vi "Test Test Unit API.vi"() -> ()   [LabVIEW 2025]
doc: "Test Unit API Tester."
uses:
  Test Unit.lvlib
  <vilib>/Utility/error.llb/DialogType.ctl
  <vilib>/Test Bench Framework/Test Executive.lvlibp/TestEngine/TestEngine/TestEngine/Report Format.ctl
  <vilib>/Test Bench Framework/Test Executive.lvlibp/TestEngine/TestEngine/TestEngine/Test Engine.lvclass
  <vilib>/Test Bench Framework/Test Executive.lvlibp/TestEngine/TestEngine/TestEngine/Typedefs/Local Report Configuration.ctl
  <vilib>/Test Bench Framework/Test Executive.lvlibp/TestEngine/TestEngine/TestEngine/Typedefs/Database Configuration.ctl
  <vilib>/Test Bench Framework/Test Executive.lvlibp/TestEngine/TestEngine/TestEngine/Typedefs/TestEngine Cofiguration.ctl
panel:
  in  "LanguageChanged":bool
  in  "Tab Control":T1(tab)
  in  "Number of socket":i32=1 min=1 max=255 step=1
  in  "TitleWindows":bool
  in  "Run New Module":bool
  in  "Select Module":i32(ring)=-1 caption="Select Module\nTo send Request to" items=["All"=-1]
  in  "Refresh Modules":bool
  in  "TestEngine Cofiguration":T2={"Break on Failure"=FALSE, "Automatically handle TestVI error"={"Enable"=FALSE, "Handle"=enum."Termination test"}, "Local Report Configuration"={"Report Folder Path"=path "D:/", "Format"=enum."CSV(,)", "Disable"=FALSE, "Build Date Folder?"=TRUE, "Execl Template Path"=path ""}, "Database Configuration"={"Connection String Expression"="", "Microsoft Data Link File"=path "", "Connection Type"=enum."Use Connection String Expression", "Enable"=FALSE}, "Ignore breakpoint"=FALSE, "Filter Result"=FALSE}
  in  "Cofiguration":bool
  in  "Load Sequence":bool
  in  "File Path Control":path
  in  "Set SN":bool
  in  "Socket":i32
  in  "Serial Number":string
  in  "Abort VI":bool=TRUE
  in  "Terminate Test":bool
  in  "Start UUTsTest":bool
  in  "Start Test":bool
  in  "Test Socket":i32
  in  "Enable Socket":bool[](array[boolean])
  in  "Set Variable":bool
  in  "Get Variable":bool
  in  "Socket(Variable)":i32
  in  "Variable Name":string
  out "Value":variant
  out "last error":errorcluster
  out "Active Modules":string[](array[string])
  in  "Stop Module":bool
  out "Status":string
  # "启动单槽位测试"
  # "启动多槽位测试"
  # "只有这个模式可以使用同步属性"
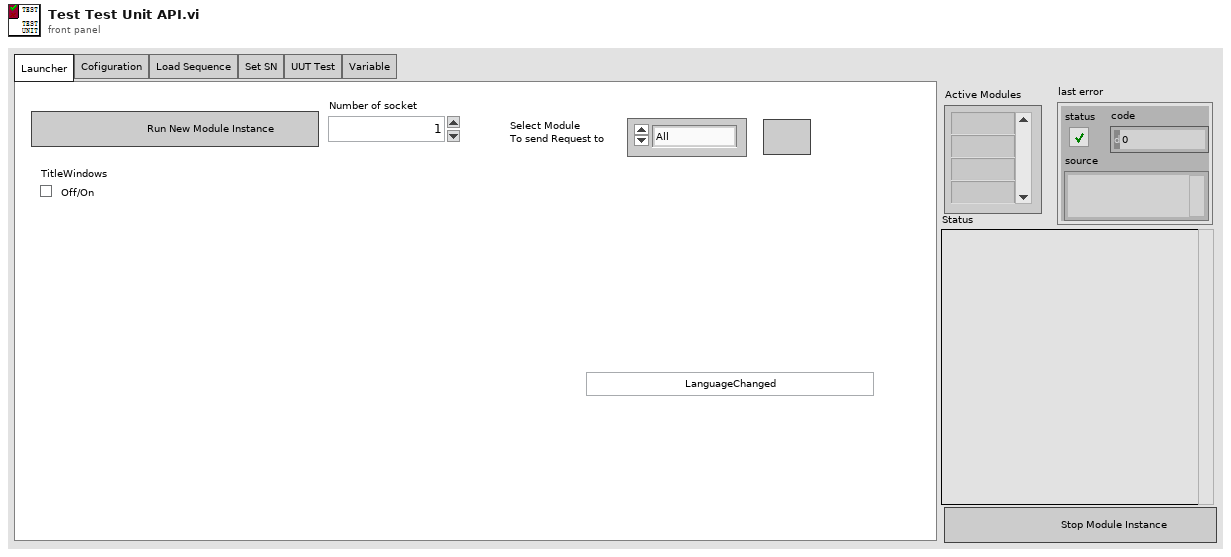
[diagram p1: front panel]
types:
  T1 = enum32{"Launcher", "Cofiguration", "Load Sequence", "Set SN", "UUT Test", "Variable"}
  T2 = typedef "Test Executive.lvlibp/Test Engine.lvlib/Test Engine.lvclass/TestEngine Cofiguration.ctl" = cluster{"Break on Failure":bool, "Automatically handle TestVI error":cluster{"Enable":bool, "Handle":enum16{"Termination test", "Ignore error"}}, "Local Report Configuration":T3, "Database Configuration":T5, "Ignore breakpoint":bool, "Filter Result":bool}
  T3 = typedef "Test Executive.lvlibp/Test Engine.lvlib/Test Engine.lvclass/Local Report Configuration.ctl" = cluster{"Report Folder Path":path, "Format":T4, "Disable":bool, "Build Date Folder?":bool, "Execl Template Path":path}
  T4 = typedef "Test Executive.lvlibp/Test Engine.lvlib/Test Engine.lvclass/Report Format.ctl" = enum16{"Excel", "CSV(Tab)", "CSV(,)", "CSV(;)", "TEXT", "HTML"}
  T5 = typedef "Test Executive.lvlibp/Test Engine.lvlib/Test Engine.lvclass/Database Configuration.ctl" = cluster{"Connection String Expression":string, "Microsoft Data Link File":path, "Connection Type":enum16{"Use Connection String Expression", "Use Microsoft Data Link File"}, "Enable":bool}
  T6 = typedef "Test Unit.lvlib/Broadcast Events--cluster.ctl" = cluster{"Module Did Init":refnum<user-event>, "Status Updated":refnum<user-event>, "Error Reported":refnum<user-event>, "Module Did Stop":refnum<user-event>, "Update Module Execution Status":refnum<user-event>}
  T7 = typedef "DialogType.ctl" = u16
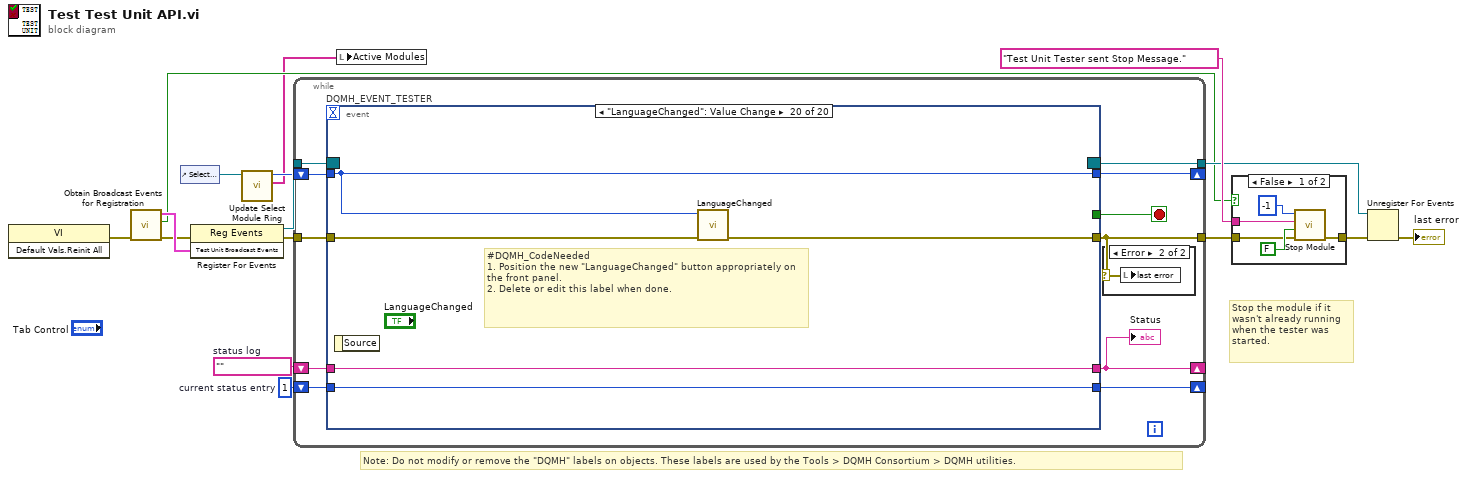
[diagram p0: block diagram]
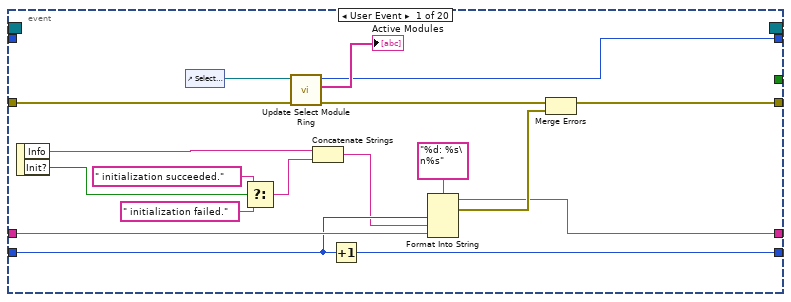
[diagram p4: hidden frame]
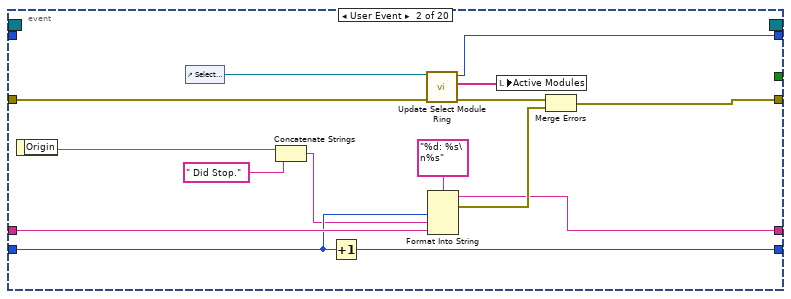
[diagram p5: hidden frame]
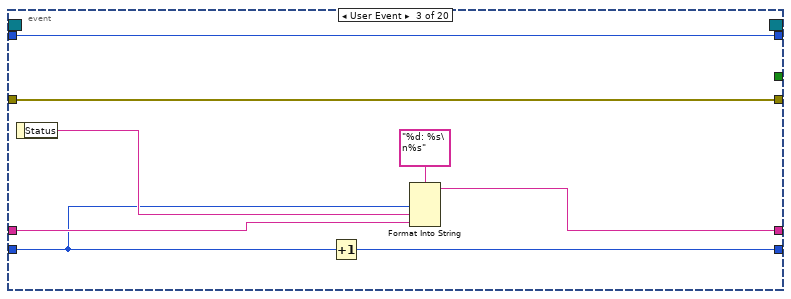
[diagram p6: hidden frame]
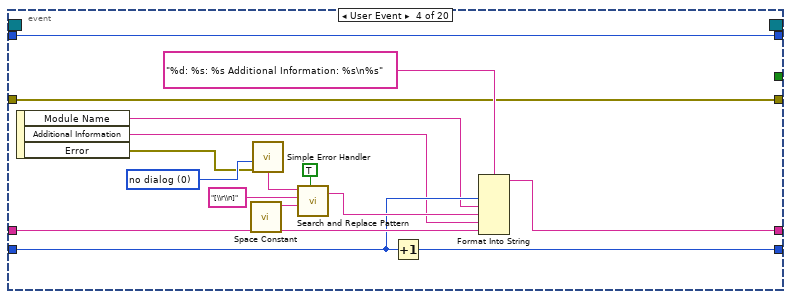
[diagram p7: hidden frame]
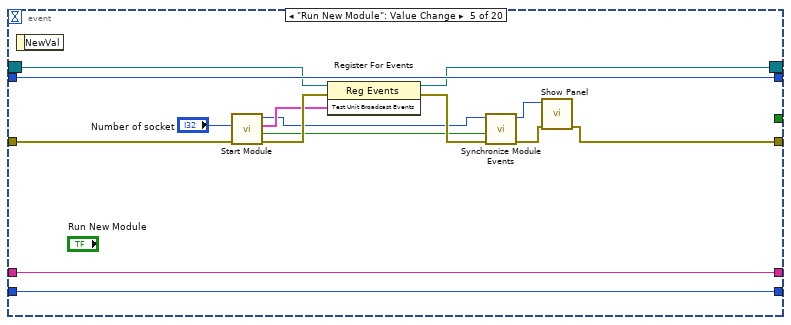
[diagram p8: hidden frame]
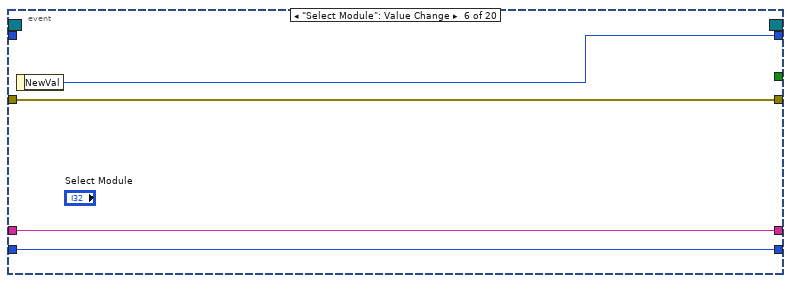
[diagram p9: hidden frame]
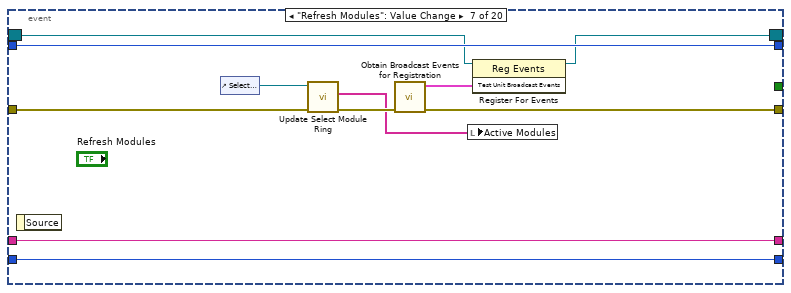
[diagram p10: hidden frame]
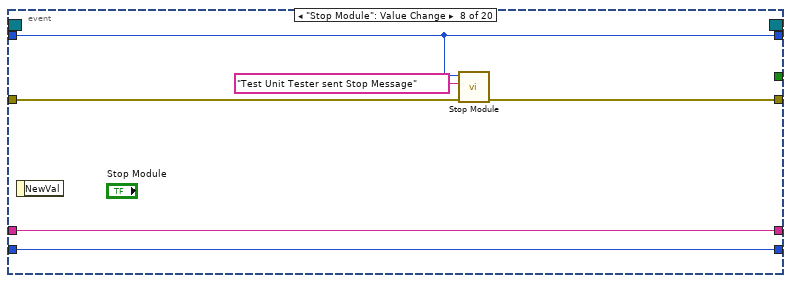
[diagram p11: hidden frame]
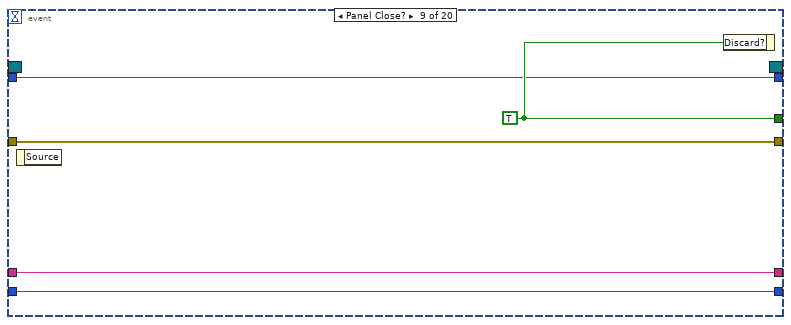
[diagram p12: hidden frame]
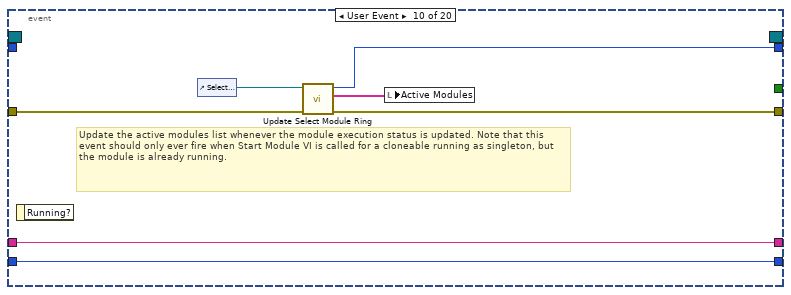
[diagram p13: hidden frame]
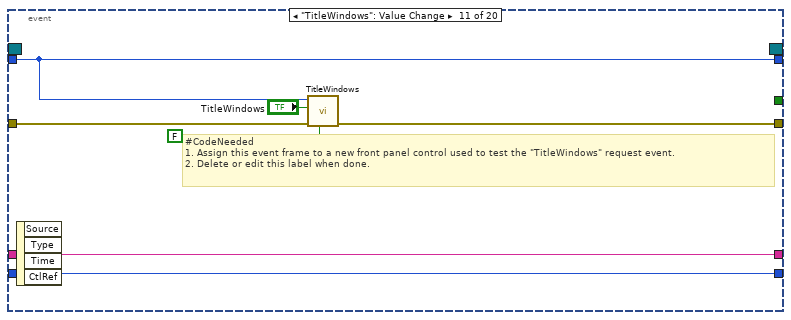
[diagram p14: hidden frame]
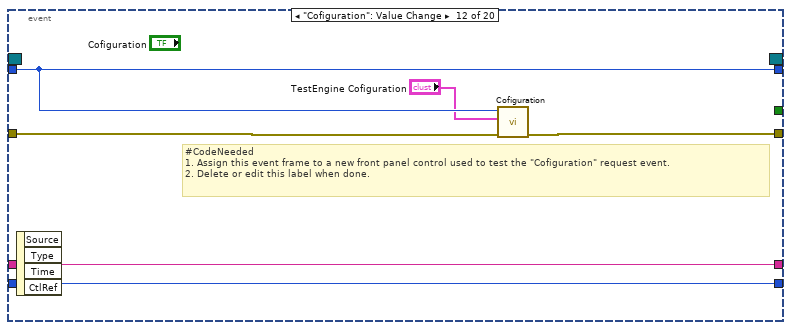
[diagram p15: hidden frame]
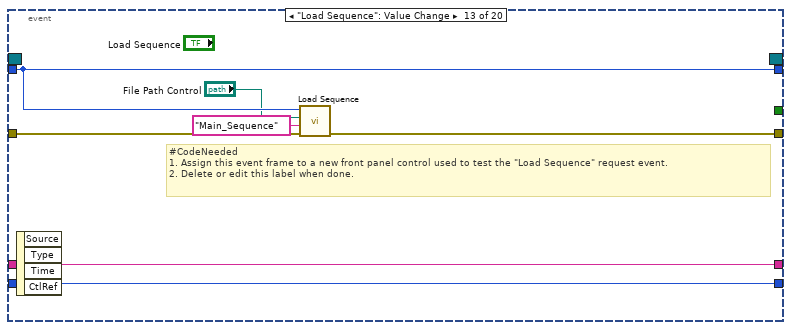
[diagram p16: hidden frame]
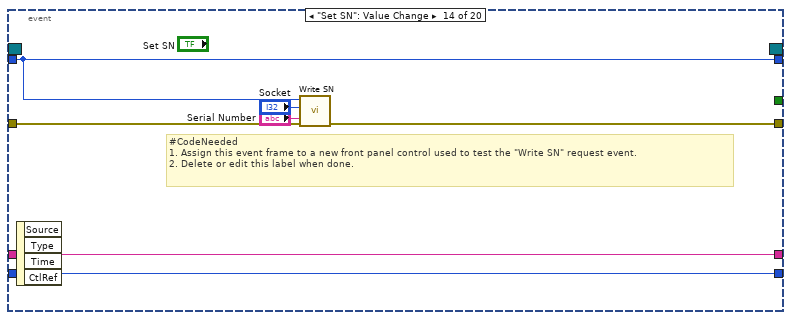
[diagram p17: hidden frame]
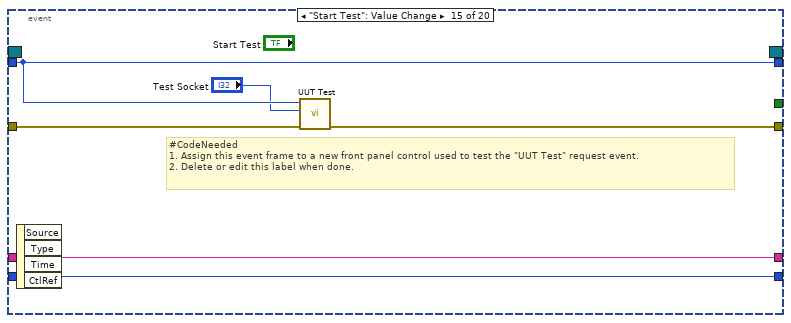
[diagram p18: hidden frame]
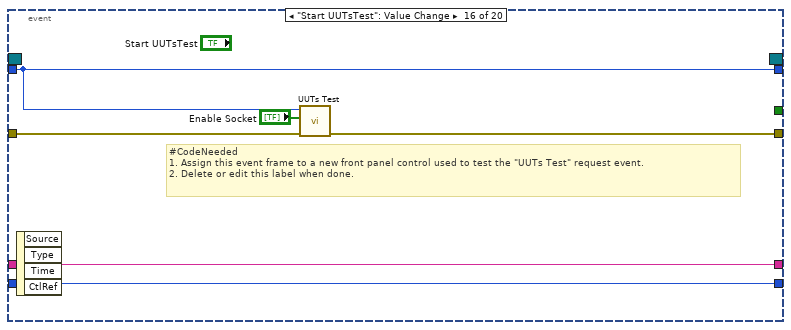
[diagram p19: hidden frame]
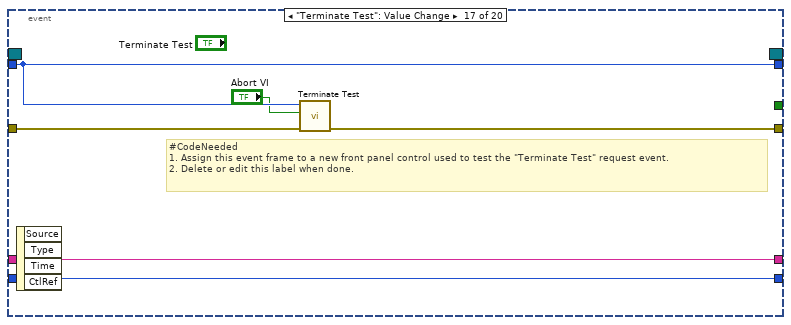
[diagram p20: hidden frame]
diagram:
  w13 = 1  # current status entry
  w14 = ""  # status log
  # "Stop the module if it wasn't already running when the tester was started."
  # "Note: Do not modify or remove the \"DQMH\" labels on objects. These labels are used by the Tools > DQMH Consortium > DQMH utilities."
  n1 = invoke class="VI" method="Default Vals.Reinit All"() -> (error out=w8:errorcluster)  [unwired: 3 in, 2 out]
  n2 = call "Obtain Broadcast Events for Registration.vi"("error in"=w8) -> ("error out"=w7:errorcluster, "Already running?"=w6:bool, "Test Unit Broadcast Events"=w12:T6)  [unwired: 8 in]
  n3 = control-ref of="Select Module"() -> (w3:refnum<vi>)
  n4 = register-events(error in=w7, w12) -> (reference out=w16:refnum<event-registration>, error out=w11:errorcluster)  [unwired: 1 in]
  n5 = call "Update Select Module Ring.vi"("Select Module Ring Ref"=w3) -> ("Active Modules (Array)"=w1:string[], "New Module Ring Value"=w2:i32)  [unwired: 8 in, 1 out]
  n6 = while {
    tunnel: w16 -> [w27]
    tunnel: [w18] -> w5
    tunnel: w11 -> [w26]
    shift-right: [w22] -> _
    shift-left: w14 -> [w24]
    shift-right: [w23] -> _
    shift-left: w13 -> [w25]
    shift-right: [w20] -> _
    shift-left: w2 -> [w21]
    tunnel: [w19] -> w9
    stop <- w17 stop-if-true
    n7 = event "DQMH_EVENT_TESTER" shown="[19] \"LanguageChanged\": Value Change" {
      selector: w27 -> [_ _ _ _ w94 _ w110 _ _ _ _ _ _ _ _ _ _ _ _ _]
      dyn-events: [_ _ _ _ w93 _ w109 _ _ _ _ _ _ _ _ _ _ _ _ _] -> w19
      timeout: _ -> [_ _ _ _ _ _ _ _ _ _ _ _ _ _ _ _ _ _ _ _]
      tunnel: [_ _ _ _ _ _ _ _ w126 _ _ _ _ _ _ _ _ _ _ _] -> w17
      tunnel: [w36 w53 w69 w73 w86 w104 w106 w117 w125 w129 w136 w142 w149 w156 w162 w168 w174 w179 w191 w196] -> w18
      tunnel: w26 -> [w38 w55 w69 w73 w95 w104 w111 w118 w125 w130 w140 w146 w153 w160 w166 w172 w178 w183 w195 w200]
      tunnel: w25 -> [w43 w58 w62 w76 w97 w102 w114 w120 w123 w132 w138 w144 w151 w158 w164 w170 w176 w181 w193 w198]
      tunnel: w24 -> [w44 w59 w65 w77 w98 w103 w115 w121 w124 w133 w139 w145 w152 w159 w165 w171 w177 w182 w194 w199]
      tunnel: [w41 w56 w66 w75 w98 w103 w115 w121 w124 w133 w139 w145 w152 w159 w165 w171 w177 w182 w194 w199] -> w22
      tunnel: [w42 w57 w68 w74 w97 w102 w114 w120 w123 w132 w138 w144 w151 w158 w164 w170 w176 w181 w193 w198] -> w23
      tunnel: w21 -> [_ _ w63 w85 w96 _ w113 w119 w122 _ w137 w143 w150 w157 w163 w169 w175 w180 w192 w197]
      tunnel: [w33 w50 w63 w85 w96 w101 w113 w119 w122 w128 w137 w143 w150 w157 w163 w169 w175 w180 w192 w197] -> w20
      event User Event {
        n8 = event-data() -> ("Info"=w40:string, "Init?"=w30:bool)  [unwired: 1 in]
        n9 = control-ref of="Select Module"() -> (w35:refnum<vi>)
        n10 = Select(t=" initialization succeeded.", s=w30, f=" initialization failed.") -> (s? t:f=w29:string)
        n11 = call "Update Select Module Ring.vi"("error in"=w38, "Select Module Ring Ref"=w35) -> ("error out"=w37:errorcluster, "Active Modules (Array)"=→"Active Modules":string[], "New Module Ring Value"=w33:i32)  [unwired: 7 in]
        n12 = Concatenate Strings(w40, w29) -> (w39:string)
        n13 = Increment(x=w43) -> (x+1=w42:i32)
        n14 = Format Into String(format string="%d: %s\n%s", w43, w39, w44) -> (resulting string=w41:string, error out=w46:errorcluster)  [unwired: 2 in]
        n15 = Merge Errors(w37, w46) -> (w36:errorcluster)
      }
      event User Event {
        n16 = event-data() -> ("Origin"=w48:string)  [unwired: 1 in]
        n17 = control-ref of="Select Module"() -> (w52:refnum<vi>)
        n18 = Concatenate Strings(w48, " Did Stop.") -> (w47:string)
        n19 = Increment(x=w58) -> (x+1=w57:i32)
        n20 = call "Update Select Module Ring.vi"("error in"=w55, "Select Module Ring Ref"=w52) -> ("error out"=w54:errorcluster, "Active Modules (Array)"=w51:string[], "New Module Ring Value"=w50:i32)  [unwired: 7 in]
        n21 = Format Into String(format string="%d: %s\n%s", w58, w47, w59) -> (resulting string=w56:string, error out=w61:errorcluster)  [unwired: 2 in]
        n22 = local write "Active Modules"(w51) -> ()
        n23 = Merge Errors(w54, w61) -> (w53:errorcluster)
      }
      event User Event {
        n24 = event-data() -> ("Status"=w64:string)  [unwired: 1 in]
        n25 = Increment(x=w62) -> (x+1=w68:i32)
        n26 = Format Into String(format string="%d: %s\n%s", w62, w64, w65) -> (resulting string=w66:string)  [unwired: 2 in, 1 out]
      }
      event User Event {
        w78 = T7 0 items=["no dialog", "OK message", "continue or stop message", "OK message + warnings", "continue/stop + warnings"] ("type of dialog (OK msg:1)")
        n27 = event-data() -> ("Module Name"=w72:string, "Additional Information"=w71:string, "Error"=w70:errorcluster)  [unwired: 1 in]
        n28 = call <vilib>:"Space Constant.vi"() -> ("String"=w82:string)
        n29 = call <vilib>:"Simple Error Handler.vi"("type of dialog (OK msg:1)"=w78, "error in (no error)"=w70) -> ("message"=w79:string)  [unwired: 3 in, 4 out]
        n30 = call <vilib>:"Search and Replace Pattern.vi"("string"=w79, "regular expression (\"\")"="[\\r\\n]" ("regular expression (\"\")"), "replace string (\"\")"=w82, "replace all? (F)"=TRUE ("replace all CR/LF with spaces")) -> ("result string"=w80:string)  [unwired: 1 in, 1 out]
        n31 = Increment(x=w76) -> (x+1=w74:i32)
        n32 = Format Into String(format string="%d: %s: %s Additional Information: %s\n%s", w76, w72, w80, w71, w77) -> (resulting string=w75:string)  [unwired: 2 in, 1 out]
      }
      event "Run New Module": Value Change {
        n33 = event-data() -> ()  [unwired: 1 in, 1 out]
        n34 = call "Start Module.vi"("error in"=w95, "Number of socket"="Number of socket") -> ("error out"=w99:errorcluster, "Wait for Event Sync?"=w92:bool, "Test Unit Broadcast Events"=w91:T6, "Module ID"=w90:i32)  [unwired: 6 in]
        n35 = register-events(reference=w94, error in=w99, w91) -> (reference out=w93:refnum<event-registration>, error out=w100:errorcluster)
        n36 = call "Synchronize Module Events.vi"("error in"=w100, "Wait for Event Sync?"=w92, "Module ID in"=w90) -> ("error out"=w87:errorcluster, "Module ID out"=w88:i32)  [unwired: 7 in]
        n37 = call "Show Panel.vi"("error in"=w87, "Module ID"=w88) -> ("error out"=w86:errorcluster)  [unwired: 9 in]
      }
      event "Select Module": Value Change {
        n38 = event-data() -> ("NewVal"=w101:i32)  [unwired: 1 in]
      }
      event "Refresh Modules": Value Change {
        n39 = event-data() -> ()  [unwired: 1 in, 1 out]
        n40 = control-ref of="Select Module"() -> (w112:refnum<vi>)
        n41 = call "Update Select Module Ring.vi"("error in"=w111, "Select Module Ring Ref"=w112) -> ("error out"=w107:errorcluster, "Active Modules (Array)"=w105:string[])  [unwired: 7 in, 1 out]
        n42 = call "Obtain Broadcast Events for Registration.vi"("error in"=w107) -> ("error out"=w106:errorcluster, "Test Unit Broadcast Events"=w108:T6)  [unwired: 8 in, 1 out]
        n43 = local write "Active Modules"(w105) -> ()
        n44 = register-events(reference=w110, w108) -> (reference out=w109:refnum<event-registration>)  [unwired: 1 in, 1 out]
      }
      event "Stop Module": Value Change {
        n45 = event-data() -> ()  [unwired: 1 in, 1 out]
        n46 = call "Stop Module.vi"("error in"=w118, "Origin"="Test Unit Tester sent Stop Message", "Module ID"=w119) -> ("error out"=w117:errorcluster)  [unwired: 8 in]
      }
      event Panel Close? {
        w126 = TRUE ("Discard?")
        n47 = event-data() -> ()  [unwired: 1 in, 1 out]
        n48 = event-data("Discard?"=w126) -> ()  [unwired: 1 in, 1 out]
      }
      event User Event {
        # "Update the active modules list whenever the module execution status is updated. Note that this event should only ever fire when Start Module VI is called for a cloneable running as singleton, but the module is already running."
        n49 = event-data() -> ()  [unwired: 1 in, 1 out]
        n50 = control-ref of="Select Module"() -> (w131:refnum<vi>)
        n51 = call "Update Select Module Ring.vi"("error in"=w130, "Select Module Ring Ref"=w131) -> ("error out"=w129:errorcluster, "Active Modules (Array)"=w127:string[], "New Module Ring Value"=w128:i32)  [unwired: 7 in]
        n52 = local write "Active Modules"(w127) -> ()
      }
      event "TitleWindows": Value Change {
        # "#CodeNeeded\n1. Assign this event frame to a new front panel control used to test the \"TitleWindows\" request event.\n2. Delete or edit this label when done."
        n53 = event-data() -> ()  [unwired: 1 in, 4 out]
        n54 = call "TitleWindows.vi"("dont initi"=FALSE, "error in"=w140, "TitleWindows"="TitleWindows", "Module ID"=w137) -> ("error out"=w136:errorcluster)  [unwired: 7 in]
      }
      event "Cofiguration": Value Change {
        # "#CodeNeeded\n1. Assign this event frame to a new front panel control used to test the \"Cofiguration\" request event.\n2. Delete or edit this label when done."
        n55 = event-data() -> ()  [unwired: 1 in, 4 out]
        n56 = call "Cofiguration.vi"("error in"=w146, "TestEngine Cofiguration"="TestEngine Cofiguration", "Module ID"=w143) -> ("error out"=w142:errorcluster)  [unwired: 8 in]
      }
      event "Load Sequence": Value Change {
        # "#CodeNeeded\n1. Assign this event frame to a new front panel control used to test the \"Load Sequence\" request event.\n2. Delete or edit this label when done."
        n57 = event-data() -> ()  [unwired: 1 in, 4 out]
        n58 = call "Load Sequence.vi"("error in"=w153, "Sequence"="Main_Sequence", "Config"="File Path Control", "Module ID"=w150) -> ("error out"=w149:errorcluster)  [unwired: 7 in]
      }
      event "Set SN": Value Change {
        # "#CodeNeeded\n1. Assign this event frame to a new front panel control used to test the \"Write SN\" request event.\n2. Delete or edit this label when done."
        n59 = event-data() -> ()  [unwired: 1 in, 4 out]
        n60 = call "Write SN.vi"("error in"=w160, "Serial Number"="Serial Number", "Socket"="Socket", "Station ID"=w157) -> ("error out"=w156:errorcluster)  [unwired: 7 in]
      }
      event "Start Test": Value Change {
        # "#CodeNeeded\n1. Assign this event frame to a new front panel control used to test the \"UUT Test\" request event.\n2. Delete or edit this label when done."
        n61 = event-data() -> ()  [unwired: 1 in, 4 out]
        n62 = call "UUT Test.vi"("error in"=w166, "Socket"="Test Socket", "Station ID"=w163) -> ("error out"=w162:errorcluster)  [unwired: 8 in]
      }
      event "Start UUTsTest": Value Change {
        # "#CodeNeeded\n1. Assign this event frame to a new front panel control used to test the \"UUTs Test\" request event.\n2. Delete or edit this label when done."
        n63 = event-data() -> ()  [unwired: 1 in, 4 out]
        n64 = call "UUTs Test.vi"("error in"=w172, "Enable Socket"="Enable Socket", "Station ID"=w169) -> ("error out"=w168:errorcluster)  [unwired: 8 in]
      }
      event "Terminate Test": Value Change {
        # "#CodeNeeded\n1. Assign this event frame to a new front panel control used to test the \"Terminate Test\" request event.\n2. Delete or edit this label when done."
        n65 = event-data() -> ()  [unwired: 1 in, 4 out]
        n66 = call "Terminate Test.vi"("error in"=w178, "Abort VI"="Abort VI", "Station ID"=w175) -> ("error out"=w174:errorcluster)  [unwired: 8 in]
      }
      event "Set Variable": Value Change {
        # "#CodeNeeded\n1. Assign this event frame to a new front panel control used to test the \"Set Variable\" request event.\n2. Delete or edit this label when done."
        n67 = event-data() -> ()  [unwired: 1 in, 4 out]
        n68 = disable-structure shown="Disabled" {
          disable-tunnel: w183 -> [w186 w187]
          disable-tunnel: w180 -> [w185 _]
          disable-tunnel: [w184 w187] -> w179
          frame Disabled {
            n69 = call "Set Variable.vi"("error in"=w186, "Station ID"=w185) -> ("error out"=w184:errorcluster)  [unwired: 9 in]
          }
          frame Enabled {
          }
        }
      }
      event "Get Variable": Value Change {
        # "#CodeNeeded\n1. Assign this event frame to a new front panel control used to test the \"Get Variable\" request event.\n2. Delete or edit this label when done."
        n70 = event-data() -> ()  [unwired: 1 in, 4 out]
        n71 = call "Get Variable.vi"("error in"=w195, "Variable"="Variable Name", "Socket"="Socket(Variable)", "Station ID"=w192) -> ("error out"=w191:errorcluster, "Value"=→"Value":variant)  [unwired: 3 in, 3 out]
      }
      event "LanguageChanged": Value Change {
        # "#DQMH_CodeNeeded\n1. Position the new \"LanguageChanged\" button appropriately on the front panel.\n2. Delete or edit this label when done."
        n72 = event-data() -> ()  [unwired: 1 in, 1 out]
        n73 = call "LanguageChanged.vi"("error in"=w200, "Module ID"=w197) -> ("error out"=w196:errorcluster)  [unwired: 9 in]
      }
    }
    "Status" <- w22
    n74 = case shown="Error" w18 {
      selector: w18 -> [_ w28]
      frame No Error {
      }
      frame Error {
        n75 = local write "last error"(w28) -> ()
      }
    }
  }
  n76 = local write "Active Modules"(w1) -> ()
  n77 = case shown="False" w6 {
    tunnel: [w205 w206] -> w15
    tunnel: "Test Unit Tester sent Stop Message." ("Origin") -> [w204 _]
    tunnel: w5 -> [w201 w206]
    frame False {
      n78 = call "Stop Module.vi"("error in"=w201, "Wait for Module to stop? (F)"=FALSE ("Wait for Module to stop?"), "Origin"=w204, "Module ID"=-1 ("Stop all")) -> ("error out"=w205:errorcluster)  [unwired: 7 in]
    }
    frame True {
    }
  }
  n79 = Unregister For Events(event registration refnum=w9, error in=w15) -> (error out=→"last error":errorcluster)
